vi "Validate Channels.vi"(10 "Channel Paths":string[](array[string]), 11 "Root":refnum<k24>) -> (3 "Valid Channels?":bool)   [LabVIEW 2013, in "Workspace MultiY Graph.lvlib"]
uses:
  Workspace MultiY Graph.lvlib
  NationalInstruments.VeriStand.SystemStorage
  NationalInstruments.VeriStand
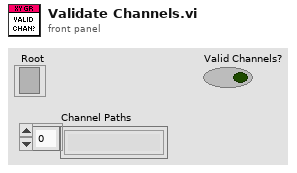
[diagram p1: front panel]
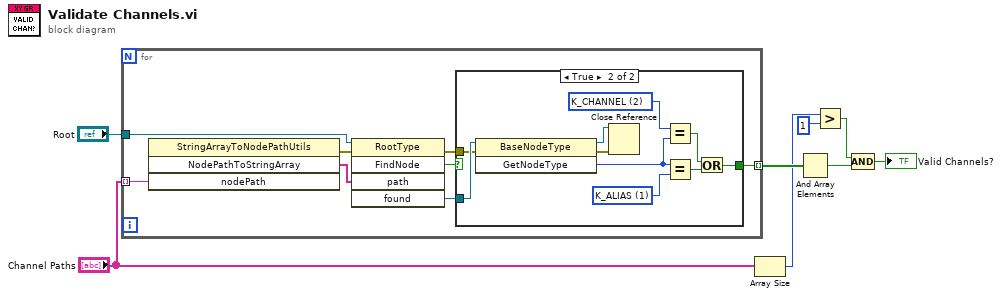
[diagram p0: block diagram]
diagram:
  n1 = for {
    tunnel: "Channel Paths" -> [w13] mode=indexing
    tunnel: "Root" -> [w14]
    tunnel: [w10] -> w6 mode=indexing
    n2 = invoke class="StringArrayToNodePathUtils" method="NodePathToStringArray"("nodePath"=w13) -> (error out=w16:errorcluster, "NodePathToStringArray"=w15:string[])  [unwired: 3 in, 2 out]
    n3 = invoke class="RootType" method="FindNode"(reference=w14, error in=w16, "path"=w15) -> (error out=w9:errorcluster, "FindNode"=w12:bool, "found"=w11:refnum<k24>)  [unwired: 2 in, 2 out]
    n4 = case shown="True" w12 {
      selector: w12 -> [w17 _]
      tunnel: w11 -> [_ w27]
      tunnel: [w17 w20] -> w10
      tunnel: w9 -> [_ w26]
      frame False {
      }
      frame True {
        w23 = 1 items=["K_BASE", "K_ALIAS", "K_CHANNEL", "K_SECTION", "K_TARGET", "K_TARGETSECTION", "K_ROOT", "K_WAVEFORM"] ("GetNodeType")
        w19 = 2 items=["K_BASE", "K_ALIAS", "K_CHANNEL", "K_SECTION", "K_TARGET", "K_TARGETSECTION", "K_ROOT", "K_WAVEFORM"] ("GetNodeType")
        n5 = invoke class="BaseNodeType" method="GetNodeType"(reference=w27, error in=w26) -> (reference out=w24:refnum<k24>, error out=w25:errorcluster, "GetNodeType"=w18:i32)  [unwired: 1 in]
        n6 = Close Reference(reference=w24, error in (no error)=w25) -> ()  [unwired: 1 out]
        n7 = Equal?(x=w19, y=w18) -> (x = y?=w22:bool)
        n8 = Equal?(x=w18, y=w23) -> (x = y?=w21:bool)
        n9 = Or(x=w22, y=w21) -> (x .or. y?=w20:bool)
      }
    }
  }
  n10 = Array Size(array="Channel Paths") -> (size(s)=w4:i32)
  n11 = And Array Elements(Boolean array=w6) -> (logical AND=w2:bool)
  n12 = Greater?(x=w4, y=1) -> (0:w3:bool)
  n13 = Compound Arithmetic op=AND(w3, w2) -> (→"Valid Channels?":bool)
